vi "Read outputs.vi"(9 "TestCase in":refnum<class "TestCase.lvclass">) -> (3 "TestCase out":refnum<class "TestCase.lvclass">, 4 "outputs":string[](array[string]))   [LabVIEW 2014, in "TestCase.lvclass"]
uses:
  TestCase.lvclass
  TestCase.lvclass/TestCase.ctl
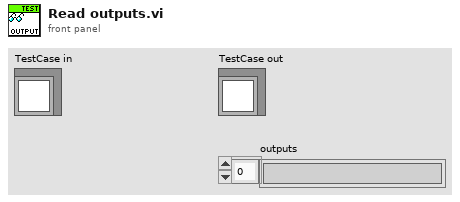
[diagram p1: front panel]
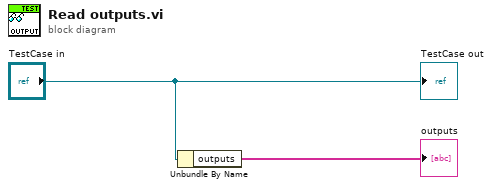
[diagram p0: block diagram]
diagram:
  n1 = Unbundle By Name("TestCase in") -> ("outputs"=→"outputs":string[])
  "TestCase out" <- "TestCase in"
